vi "XLP80_Action_WriteStreamItems.vi"(4 "TDefPath FCE1":path=path "B:/Kirschenhofer/FutureE/FCE1/Software/01_SourceCode/FCE1_ProjectLibs", 8 "error in":errorcluster) -> (0 "error out":errorcluster)   [LabVIEW 2021]
uses:
  XLP80_FGlob/XLP80_FGlob_TDefEnumcDAQAIItems.ctl
  XLP80_FGlob/XLP80_FGlob_TDefEnumcDAQAOItems.ctl
  XLP80_FGlob/XLP80_FGLob_TDefEnumCalcAnalogItems.ctl
panel:
  in  "CalculatedValues_Items":T1
  in  "PCI AO Item":T2
  in  "PCI AI Item":T3
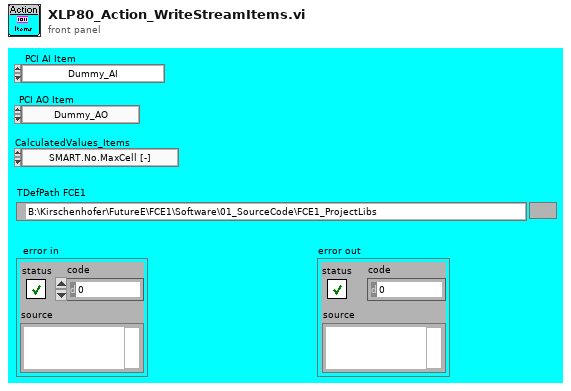
[diagram p1: front panel]
types:
  T1 = typedef "XLP80_FGLob_TDefEnumCalcAnalogItems.ctl" = enum8{"SMART.No.MaxCell [-]", "SMART.No.MinCell [-]", "SMART.U.S.AveCell [V]", "SMART.U.S.CVM [V]", "SMART.U.S.MaxCell [V]", "SMART.U.S.MinCell [V]"}
  T2 = typedef "XLP80_FGlob_TDefEnumcDAQAOItems.ctl" = enum16{"Dummy_AO"}
  T3 = typedef "XLP80_FGlob_TDefEnumcDAQAIItems.ctl" = enum16{"Dummy_AI"}
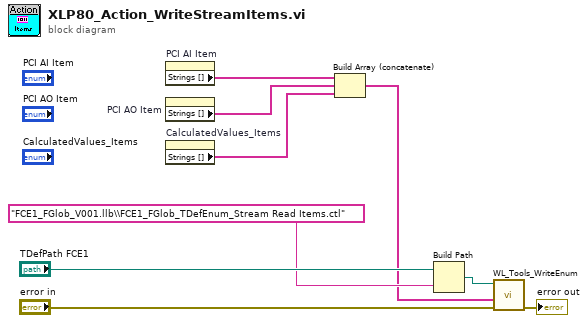
[diagram p0: block diagram]
diagram:
  n1 = property on="PCI AI Item" class="Enum (strict)"() -> ("Strings []"=w4:string[])  [unwired: 2 in, 2 out]
  n2 = property on="PCI AO Item" class="Enum (strict)"() -> ("Strings []"=w3:string[])  [unwired: 2 in, 2 out]
  n3 = property on="CalculatedValues_Items" class="Enum (strict)"() -> ("Strings []"=w2:string[])  [unwired: 2 in, 2 out]
  n4 = Build Array (concatenate)(w4, w3, w2) -> (w1:string[])
  n5 = Build Path(base path="TDefPath FCE1", name or relative path="FCE1_FGlob_V001.llb\\FCE1_FGlob_TDefEnum_Stream Read Items.ctl" ("string")) -> (appended path=w6:path)
  n6 = call "WL_Tools_WriteEnum.vi"("err in"="error in", "Strings"=w1, "BasePath"=w6) -> ("err out"=→"error out":errorcluster)  [unwired: 8 in]
